vi "Complex Sylvester Equations.vi"(4 "matrix type":i32(ring)=3 items=["General"=0, "Upper Triangular"=3], 6 "operation B":u16(ring) items=["Not Tranposed", "Transposed"], 7 "operation A":u16(ring) items=["Not Transposed", "Transposed"], 8 "sign":u16(ring) items=["Plus", "Minus"], 9 "C":T1, 10 "B":T1, 11 "A":T1) -> (0 "error":i32, 1 "perturbed":bool, 2 "scale":dbl=1.0, 3 "X":T1)   [LabVIEW 2020, in "NI_AALPro.lvlib"]
doc: "Solves the Sylvester matrix equation. The data types you wire to the <B>A</B>, <B>B</B>, and <B>C</B> inputs determine the polymorphic instance to use."
uses:
  NI_AALPro.lvlib
  ComplexMatrix.ctl
  <resource>/lvanlys.dll
  NI_Matrix.lvlib
panel:
  # "Solve Sylvester's Equations"
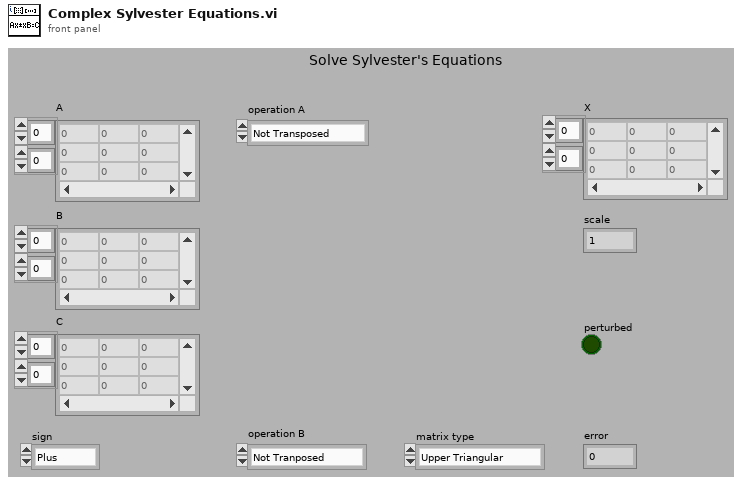
[diagram p1: front panel]
types:
  T1 = typedef "NI_Matrix.lvlib/ComplexMatrix.ctl" = cdb[][]
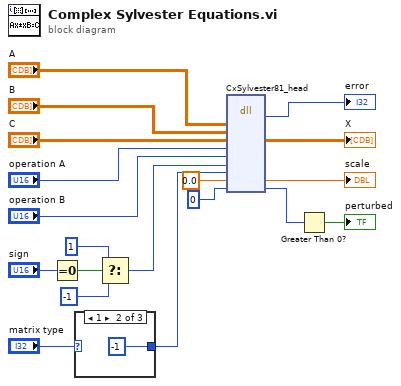
[diagram p0: block diagram]
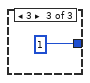
[diagram p3: hidden frame]
diagram:
  n1 = Equal To 0?(x="sign") -> (x = 0?=w11:bool)
  n2 = case shown="1" "matrix type" {
    selector: "matrix type" -> [w20 _ _]
    tunnel: [w20 -1 ("matrix type") 1] -> w2
    frame 0, Default {
    }
    frame 1 {
    }
    frame 3 {
    }
  }
  n3 = Select(t=1, s=w11, f=-1) -> (s? t:f=w8:i32)
  n4 = dll-call lib="C:/Program Files (x86)/National Instruments/LabVIEW 2020/resource/lvanlys.*" fn="CxSylvester81_head"("A"="A", "B"="B", "C"="C", "opA"="operation A", "opB"="operation B", "sgn"=w8, "type"=w2, "scale"=0.0, "perturbed"=0) -> (→"error":i32, "C"=→"X":T1, "scale"=→"scale":dbl, "perturbed"=w6:i32)  [unwired: 9 in, 2 out]
  n5 = Greater Than 0?(x=w6) -> (x > 0?=→"perturbed":bool)
